vi "START EDIT ITEMS.vi"(10 "USER/ITEM DATA TRANSFER":T2(array[cluster]), 11 "REFERENCES":T3) -> (2 "BYU ID #":string, 3 "Data Out":T1[](array[typedef]))   [LabVIEW 2019]
uses:
  Controls/References Cluster.ctl
  <vilib>/userDefined/High Color/IMAQdx.ctl
  Controls/Custom Calendar/Custom Calendar.xctl
  Controls/Table Data Types/Inventory Data Type.ctl
  <vilib>/Utility/miscctls.llb/LVRowAndColumnTypeDef.ctl
  <vilib>/addons/database/Connection.llb/DB Tools Open Connec (String).vi
  <vilib>/addons/database/_DB Variant To Data/Database Variant To Data.xnode
  <vilib>/addons/database/NI_Database_API.lvlib
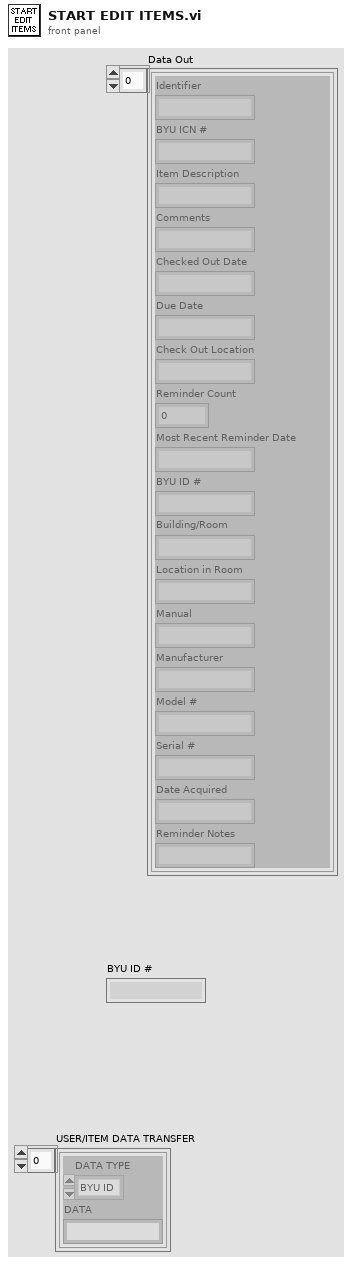
[diagram p1: front panel]
types:
  T1 = typedef "Inventory Data Type.ctl" = cluster{"Identifier":string, "BYU ICN #":string, "Item Description":string, "Comments":string, "Checked Out Date":string, "Due Date":string, "Check Out Location":string, "Reminder Count":i32, "Most Recent Reminder Date":string, "BYU ID #":string, "Building/Room":string, "Location in Room":string, "Manual":string, "Manufacturer":string, "Model #":string, "Serial #":string, "Date Acquired":string, "Reminder Notes":string}
  T2 = cluster{"DATA TYPE":enum16{"BYU ID", "ME#/IDENTIFIER", "BYU ICN"}, "DATA":string}[]
  T3 = typedef "References Cluster.ctl" = cluster{"MAIN PAGES":refnum<vi>, "ADD/EDIT ITEM REFERENCES":cluster{"Identifier":refnum<vi>, "BYU ICN #":refnum<vi>, "Item Description":refnum<vi>, "Comments":refnum<vi>, "Checked Out Date":refnum<vi>, "Due Date":refnum<vi>, "Check Out Location":refnum<vi>, "Reminder Count":refnum<vi>, "Most Recent Reminder Date":refnum<vi>, "BYU ID #":refnum<vi>, "Building/Room":refnum<vi>, "Location in Room":refnum<vi>, "Manual":refnum<vi>, "Manufacturer":refnum<vi>, "Model #":refnum<vi>, "Serial #":refnum<vi>, "Date Acquired":refnum<vi>, "ADD/EDIT ITEM LABEL":refnum<vi>, "ARCHIVE ITEM":refnum<vi>, "Archive Item Inputs":refnum<vi>, "Reminder Notes":refnum<vi>, "DUPLICATE ITEM":refnum<vi>}, "ADD/EDIT USER REFERENCES":cluster{"BYU ID # (##-###-####)":refnum<vi>, "First Name":refnum<vi>, "Last Name":refnum<vi>, "Phone Number (###-###-####)":refnum<vi>, "Email":refnum<vi>, "Department":refnum<vi>, "Graduation Status":refnum<vi>, "Anticipated Graduation Year":refnum<vi>, "Credit Score":refnum<vi>, "Date Added":refnum<vi>, "Graduation Clearance Date":refnum<vi>, "Picture File Name":refnum<vi>, "ADD/EDIT USER LABEL":refnum<vi>, "Department Map":refnum<vi>, "Status Map":refnum<vi>, "Anticipated Graduation Year Map":refnum<vi>, "User Agreement":refnum<vi>, "User Comments":refnum<vi>, "Camera":refnum<vi>}, "RETURN ITEM REFERENCES":cluster{"Item or Person:":refnum<vi>, "Search Return Results":refnum<vi>, "What are you searching for?":refnum<vi>}, "SEARCH DATABASE REFERENCES":cluster{"What to Search For:":refnum<vi>, "Where to Search":refnum<vi>, "Column to Search In":refnum<vi>, "Column to Sort By":refnum<vi>, "Search Database Results":refnum<vi>, "Inventory Column Selector":refnum<vi>, "User Column Selector":refnum<vi>, "Inventory Archive Column Selector":refnum<vi>, "User Archive Column Selector":refnum<vi>, "Sales Tracking Column Selector":refnum<vi>, "Checked In Archive Column Selector":refnum<vi>, "Restore User":refnum<vi>, "Date Range":refnum<vi>, "Dates Less Than":refnum<vi>, "Dates Greater Than":refnum<vi>, "Search Print Receipt":refnum<vi>, "Edit Sale Description":refnum<vi>}, "USER ITEMS REFERENCES":cluster{"USER'S INFORMATION":refnum<vi>, "User's Checked Out Items":refnum<vi>, "User Info Comments":refnum<vi>, "SEE USER INFO COMMENTS":refnum<vi>}, "EDIT ITEMS REFERENCES":cluster{"New Check Out Location":refnum<vi>, "Items to Edit":refnum<vi>, "Edit Items Due Date":refnum<vi>, "New Reminder Notes":refnum<vi>, "New Item Description":refnum<vi>}, "CHECK OUT ITEMS REFERENCES":cluster{"Enter Item:":refnum<vi>, "Check Out Items Due Date":refnum<vi>, "Check Out Location":refnum<vi>, "Items to be Checked Out":refnum<vi>, "Possible Items":refnum<vi>, "Altered Item Description":refnum<vi>}, "TRANSFER ITEMS REFERENCES":cluster{"Search Parameter":refnum<vi>, "What to Match":refnum<vi>, "Matching Individuals":refnum<vi>, "Items to be Transferred":refnum<vi>}, "SETTINGS REFERENCES":cluster{"PSC Database Settings":refnum<vi>, "PSC Sales Item Spreadsheet":refnum<vi>}, "PSC SALES REFERENCES":cluster{"BYU ID CARD #":refnum<vi>, "Sale Description":refnum<vi>, "Scan or Enter Item Name":refnum<vi>, "Items to be Sold":refnum<vi>, "Grand Total":refnum<vi>, "Item List":refnum<vi>}}
  T4 = typedef "LVRowAndColumnTypeDef.ctl" = cluster{"Row":i32, "Column":i32}
  T5 = enum32{"IDLE", "ADD/EDIT USER", "ADD/EDIT ITEM", "RETURN ITEMS", "SEARCH DATABASE", "USER ITEMS", "CHECK OUT ITEMS", "EDIT ITEMS", "TRANSFER ITEMS", "PSC SALES", "ATRIUM", "INVENTORY TRACKING", "SETTINGS"}
  T6 = typedef "NI_Database_API.lvlib/Conn ObjectReference.ctl" = refnum<k1>
  T7 = cluster{"New Check Out Location":refnum<vi>, "Items to Edit":refnum<vi>, "Edit Items Due Date":refnum<vi>, "New Reminder Notes":refnum<vi>, "New Item Description":refnum<vi>}
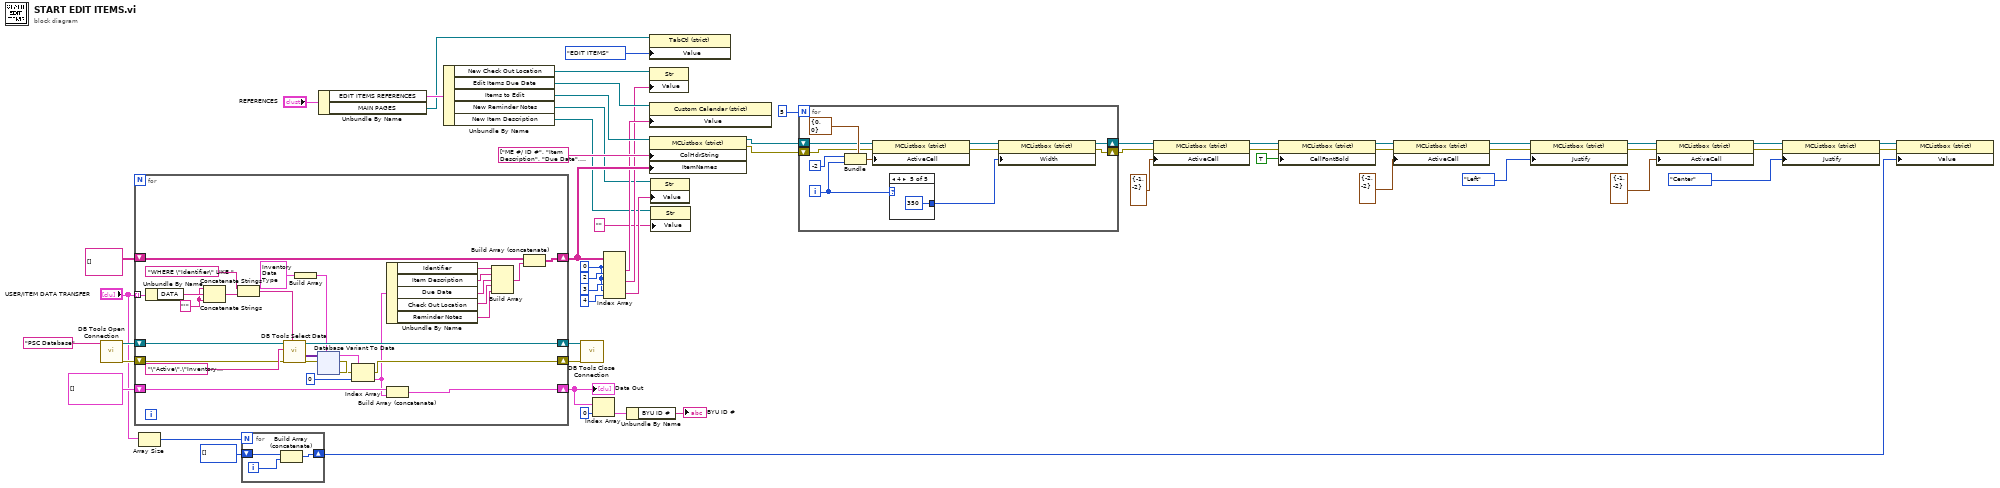
[diagram p0: block diagram]
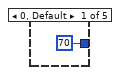
[diagram p2: hidden frame]
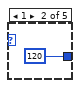
[diagram p3: hidden frame]
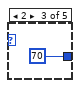
[diagram p4: hidden frame]
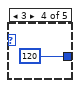
[diagram p5: hidden frame]
diagram:
  w6 = 0 ("index (row)")
  n1 = call-poly <vilib>:"DB Tools Open Connection.vi"("connection information"="PSC Database") -> ("error out"=w52:errorcluster, "connection reference"=w53:T6)  [unwired: 7 in]
  n2 = for {
    tunnel: "USER/ITEM DATA TRANSFER" -> [w81] mode=indexing
    shift-right: [w74] -> w49
    shift-left: w53 -> [w84]
    shift-right: [w75] -> w48
    shift-left: w52 -> [w83]
    shift-right: [w73] -> w40
    shift-left: T1[] [] -> [w72]
    shift-right: [w65] -> w46
    shift-left: string[][] [] -> [w64]
    w59 = "'"
    n3 = Unbundle By Name(w81) -> ("DATA"=w60:string)
    n4 = Concatenate Strings(w59, w60, w59) -> (w61:string)
    n5 = Concatenate Strings("WHERE \"Identifier\" LIKE " ("table"), w61) -> (w80:string)
    n6 = call <vilib>:"DB Tools Select Data.vi"("condition"=w80, "error in (no error)"=w83, "table"="\"Active\".\"Inventory\"", "connection reference"=w84) -> ("error out"=w79:errorcluster, "data"=w78:variant[][], "connection reference out"=w74:T6)  [unwired: 2 in]
    n7 = Build Array(T1 {"Identifier"="", "BYU ICN #"="", "Item Description"="", "Comments"="", "Checked Out Date"="", "Due Date"="", "Check Out Location"="", "Reminder Count"=0, "Most Recent Reminder Date"="", "BYU ID #"="", "Building/Room"="", "Location in Room"="", "Manual"="", "Manufacturer"="", "Model #"="", "Serial #"="", "Date Acquired"="", "Reminder Notes"=""} ("Array")) -> (w62:T1[])
    n8 = xnode "Database Variant To Data"("database variant"=w78, "error in (no error)"=w79, "type"=w62) -> ("data"=w77:T1[], "error out"=w75:errorcluster)
    n9 = Index Array(array=w77, index=0) -> (element=w71:T1)
    n10 = Unbundle By Name(w71) -> ("Identifier"=w70:string, "Item Description"=w69:string, "Due Date"=w68:string, "Check Out Location"=w67:string, "Reminder Notes"=w58:string)
    n11 = Build Array (concatenate)(w72, w71) -> (w73:T1[])
    n12 = Build Array(w70, w69, w68, w67, w58) -> (w66:string[])
    n13 = Build Array (concatenate)(w64, w66) -> (w65:string[][])
  }
  "Data Out" <- w40
  n14 = Array Size(array="USER/ITEM DATA TRANSFER") -> (size(s)=w11:i32)
  n15 = for {
    N: w11 -> [_]
    shift-right: [w654] -> w7
    shift-left: i32[] [] ("Value") -> [w656]
    i -> [w655]
    n16 = Build Array (concatenate)(w656, w655) -> (w654:i32[])
  }
  n17 = Unbundle By Name("REFERENCES") -> ("EDIT ITEMS REFERENCES"=w56:T7, "MAIN PAGES"=w36:refnum<vi>)
  n18 = Unbundle By Name(w56) -> ("New Check Out Location"=w43:refnum<vi>, "Edit Items Due Date"=w47:refnum<vi>, "Items to Edit"=w55:refnum<vi>, "New Reminder Notes"=w4:refnum<vi>, "New Item Description"=w1:refnum<vi>)
  n19 = call <vilib>:"DB Tools Close Connection.vi"("error in (no error)"=w48, "connection reference"=w49) -> ()  [unwired: 5 in, 1 out]
  n20 = Index Array(array=w40, index=0) -> (element=w38:T1)
  n21 = Index Array(array=w46, index (row) #1=w6, index (col) #1=2 ("index (row)"), index (row) #2=w6, index (col) #2=3 ("index (row)"), index (row) #3=w6, index (col) #3=4 ("index (row)")) -> (element #1=w44:string, element #2=w41:string, element #3=w3:string)
  n22 = Unbundle By Name(w38) -> ("BYU ID #"=→"BYU ID #":string)
  n23 = property class="TabCtl (strict)"(reference=w36, "Value"=T5."EDIT ITEMS") -> ()  [unwired: 1 in, 2 out]
  n24 = property class="Str"(reference=w43, "Value"=w41) -> ()  [unwired: 1 in, 2 out]
  n25 = property class="Custom Calendar (strict)"(reference=w47, "Value"=w44) -> ()  [unwired: 1 in, 2 out]
  n26 = property class="MCListbox (strict)"(reference=w55, "ColHdrString"=string[] ["ME #/ ID #", "Item Description", "Due Date", "Check Out Location", "Reminder Notes"] ("Column Header Strings[]"), "ItemNames"=w46) -> (reference out=w14:refnum<vi>, error out=w13:errorcluster)  [unwired: 1 in]
  n27 = property class="Str"(reference=w4, "Value"=w3) -> ()  [unwired: 1 in, 2 out]
  n28 = property class="Str"(reference=w1, "Value"="") -> ()  [unwired: 1 in, 2 out]
  n29 = for {
    N: 5 -> [_]
    shift-right: [w667] -> w15
    shift-left: w14 -> [w664]
    shift-right: [w666] -> w16
    shift-left: w13 -> [w663]
    i -> [w657]
    n30 = Bundle(cluster=T4 {"Row"=0, "Column"=0} ("Active Cell:Active Cell"), "Row"=-2, "Column"=w657) -> (w662:T4)
    n31 = property class="MCListbox (strict)"(reference=w664, error in=w663, "ActiveCell"=w662) -> (reference out=w660:refnum<vi>, error out=w659:errorcluster)
    n32 = case shown="4" w657 {
      tunnel: [u32 70 ("Active Cell:Cell Size:Width") u32 120 ("Active Cell:Cell Size:Width") u32 70 ("Active Cell:Cell Size:Width") u32 120 ("Active Cell:Cell Size:Width") u32 350 ("Active Cell:Cell Size:Width")] -> w658
      frame 0, Default {
      }
      frame 1 {
      }
      frame 2 {
      }
      frame 3 {
      }
      frame 4 {
      }
    }
    n33 = property class="MCListbox (strict)"(reference=w660, error in=w659, "Width"=w658) -> (reference out=w667:refnum<vi>, error out=w666:errorcluster)
  }
  n34 = property class="MCListbox (strict)"(reference=w15, error in=w16, "ActiveCell"=T4 {"Row"=-1, "Column"=-2} ("Active Cell:Active Cell")) -> (reference out=w32:refnum<vi>, error out=w31:errorcluster)
  n35 = property class="MCListbox (strict)"(reference=w32, error in=w31, "CellFontBold"=TRUE ("Active Cell:Cell Font:Bold")) -> (reference out=w29:refnum<vi>, error out=w28:errorcluster)
  n36 = property class="MCListbox (strict)"(reference=w29, error in=w28, "ActiveCell"=T4 {"Row"=-2, "Column"=-2} ("Active Cell:Active Cell")) -> (reference out=w26:refnum<vi>, error out=w25:errorcluster)
  n37 = property class="MCListbox (strict)"(reference=w26, error in=w25, "Justify"=enum16{"Left", "Center", "Right"}."Left" ("Active Cell:Cell Justification")) -> (reference out=w21:refnum<vi>, error out=w20:errorcluster)
  n38 = property class="MCListbox (strict)"(reference=w21, error in=w20, "ActiveCell"=T4 {"Row"=-1, "Column"=-2} ("Active Cell:Active Cell")) -> (reference out=w22:refnum<vi>, error out=w23:errorcluster)
  n39 = property class="MCListbox (strict)"(reference=w22, error in=w23, "Justify"=enum16{"Left", "Center", "Right"}."Center" ("Active Cell:Cell Justification")) -> (reference out=w9:refnum<vi>, error out=w8:errorcluster)
  n40 = property class="MCListbox (strict)"(reference=w9, error in=w8, "Value"=w7) -> ()  [unwired: 2 out]
